vi "Destroy.vi"(8 "Error In":errorcluster, 11 "reference in":refnum<class "SpeakTurkish.lvclass">) -> (0 "Error Out":errorcluster, 3 "reference out":refnum<class "SpeakTurkish.lvclass">)   [LabVIEW 2024, in "SpeakTurkish.lvclass"]
uses:
  SpeakTurkish.lvclass
  SpeakTurkish.lvclass/SpeakTurkish.ctl
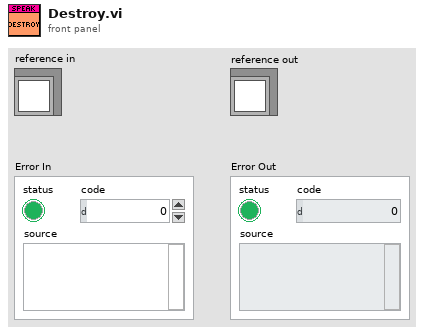
[diagram p1: front panel]
types:
  T1 = typedef "VI-TechBaseTemplate_Simple_4x4x4.lvclass/ObjectAttributes.ctl" = cluster{"Attribute1":dbl}
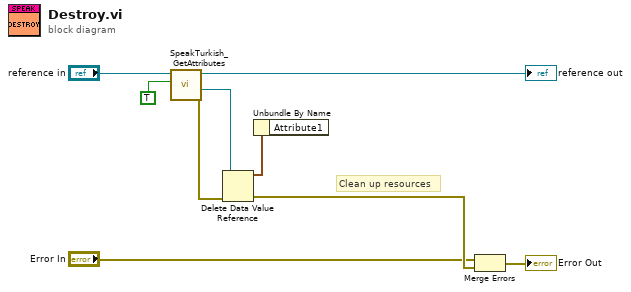
[diagram p0: block diagram]
diagram:
  # "Clean up resources"
  n1 = call "SpeakTurkish_GetAttributes.vi"("OnlyGetDvrReference(False)"=TRUE, "reference in"="reference in") -> ("Error Out"=w6:errorcluster, "DataRef"=w5:refnum<data-value>, "reference out"=→"reference out":refnum<class "SpeakTurkish.lvclass">)  [unwired: 6 in, 1 out]
  n2 = Delete Data Value Reference(data value reference=w5, error in=w6) -> (data value=w1:T1, error out=w4:errorcluster)
  n3 = Unbundle By Name(w1) -> ()  [unwired: 1 out]
  n4 = Merge Errors("Error In", w4) -> (→"Error Out":errorcluster)
